vi "Base Setup.vi"(10 "Setup":T1) -> (2 "Setup":refnum<class "Setup.lvclass">)   [LabVIEW 2025, in "jettl.lvlib" / "Setup.lvlib"]
uses:
  Setup.lvlib
  Setup/Setup.lvclass
  Setup.ctl
  Attributes/Attributes/Attributes.lvclass
  Transport/Transport/Transport.lvclass
  Msg Set.ctl
  Msg/Msg.lvclass
  Base Setup/Base Setup.lvclass
  C:/git/jettl/src/jettl/jettl/Setup/Setup/Setup.lvclass
  jettl.lvlib
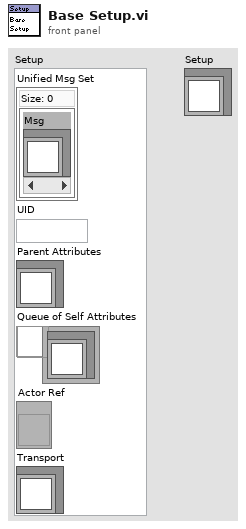
[diagram p1: front panel]
types:
  T1 = typedef "jettl.lvlib/Setup.ctl" = cluster{"Unified Msg Set":T2, "UID":string, "Parent Attributes":refnum<class "Attributes.lvclass">, "Queue of Self Attributes":refnum<queue>, "Actor Ref":refnum<vi>, "Transport":refnum<class "Transport.lvclass">}
  T2 = typedef "jettl.lvlib/Msg Set.ctl" = set{refnum<class "Msg.lvclass">}
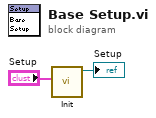
[diagram p0: block diagram]
diagram:
  n1 = call "Init.vi"("Setup"="Setup") -> ("Base Setup out"=→"Setup":refnum<class "Base Setup.lvclass">)  [unwired: 10 in]
